vi "17.3 OCR Training.vi"() -> ()   [LabVIEW 2017]
uses:
  <vilib>/vision/OCR.llb/IMAQ OCR Threshold Mode.ctl
  <vilib>/vision/OCR.llb/IMAQ OCR Property.ctl
  <vilib>/vision/NI_Vision_Development_Module.lvlib
panel:
  out "Image":T1(plugin-control)
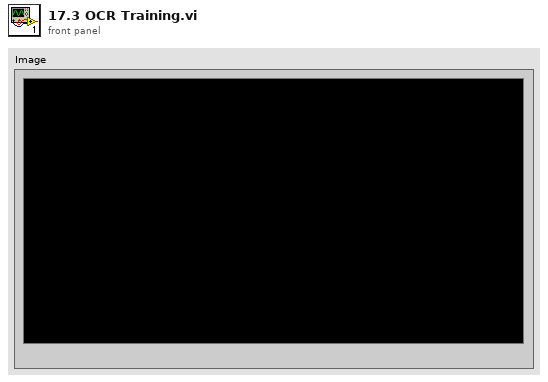
[diagram p1: front panel]
types:
  T1 = typedef "IMAQ Image.ctl" = refnum<image>
  T2 = typedef "IMAQ Rectangle" = cluster{"Left":i32, "Top":i32, "Right":i32, "Bottom":i32, "Rotation":dbl}
  T3 = typedef "IMAQ OCR Property.ctl" = i32
  T4 = cluster{"Dark Characters":bool, "Number of Blocks":i32, "Threshold Limits":cluster{"Lower Value":i32, "Upper Value":i32}, "Optimize For Speed":bool, "Perform Bi-modal Calculation":bool}
  T5 = typedef "IMAQ OCR Threshold Mode.ctl" = i32
  T6 = typedef "IMAQ OCR Session.ctl" = refnum<k1>
  T7 = typedef "ROI Descriptor" = cluster{"Global Rectangle":i32[], "Contours":cluster{"ID":enum32{"External", "Internal"}, "Type":u32, "Coordinates":i32[]}[]}
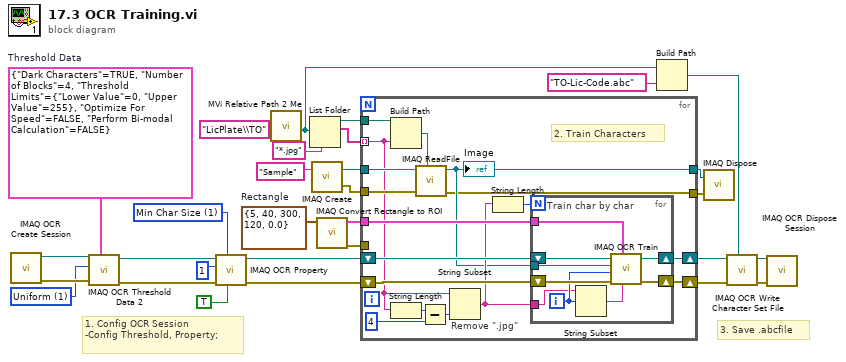
[diagram p0: block diagram]
diagram:
  w6 = T2 {"Left"=5, "Top"=40, "Right"=300, "Bottom"=120, "Rotation"=0.0}  # Rectangle
  w12 = T3 1 items=["Acceptance Level", "Min Char Size", "Max Char Size", "Min Char Spacing", "Max Horiz Element Spacing", "Max Vert Element Spacing", "Min Bounding Rect Width", "Max Bounding Rect Width", "Min Bounding Rect Height", "Max Bounding Rect Height", "Read Strategy", "Aspect Ratio", "Number Of Erosions", "Read Resolution", "Size of Char Set", "Substitution Character", "Remove Particles Touching ROI", "Auto Split", "Threshold Type", "Text Detection", "Line Separator", "Shortest Path Segment", "Min Pixels for Space"] ("Property")
  w16 = T4 {"Dark Characters"=TRUE, "Number of Blocks"=4, "Threshold Limits"={"Lower Value"=0, "Upper Value"=255}, "Optimize For Speed"=FALSE, "Perform Bi-modal Calculation"=FALSE}  # Threshold Data
  w19 = T5 1 items=["Fixed Range", "Uniform", "Linear", "Non-Linear"] ("Threshold Mode")
  # "3. Save .abcfile"
  # "1. Config OCR Session\n-Config Threshold, Property;"
  n1 = call "IMAQ OCR Create Session"() -> ("error out"=w20:errorcluster, "IMAQ OCR Session"=w21:T6)  [unwired: 10 in]
  n2 = call-poly "IMAQ OCR Threshold Data 2"("Threshold Data"=w16, "error in (no error)"=w20, "Threshold Mode"=w19, "IMAQ OCR Session"=w21) -> ("error out"=w17:errorcluster, "IMAQ OCR Session (dup)"=w18:T6)  [unwired: 3 in, 3 out]
  n3 = call-poly "IMAQ OCR Property"("Get/Set (True: Set)"=TRUE, "Property"=w12, "error in (no error)"=w17, "Property Value"=1, "IMAQ OCR Session"=w18) -> ("error out"=w15:errorcluster, "IMAQ OCR Session (dup)"=w14:T6)  [unwired: 4 in, 1 out]
  n4 = call "MVi Relative Path 2 Me.vi"("Relative Path"="LicPlate\\TO") -> ("Appended Dir"=w23:path)  [unwired: 5 in, 1 out]
  n5 = List Folder(path=w23, pattern="*.jpg") -> (path out=w25:path, filenames=w28:string[])  [unwired: 2 in, 2 out]
  n6 = call "IMAQ Create"("Image Name"="Sample") -> ("New Image"=w26:T1, "error out"=w24:errorcluster)  [unwired: 4 in]
  n7 = call "IMAQ Convert Rectangle to ROI"("Rectangle"=w6) -> ("error out"=w4:errorcluster, "ROI Descriptor"=w5:T7)  [unwired: 8 in]
  n8 = for {
    tunnel: w28 -> [w35] mode=indexing
    tunnel: w26 -> [w43]
    tunnel: w25 -> [w44]
    shift-right: [w38] -> w11
    shift-left: w15 -> [w40]
    tunnel: w24 -> [w42]
    shift-right: [w37] -> w10
    shift-left: w14 -> [w39]
    tunnel: w5 -> [w36]
    tunnel: w4 -> [_]
    tunnel: [w32] -> w2
    tunnel: [w31] -> w1
    # "2. Train Characters"
    # "Remove \".jpg\""
    n9 = Build Path(base path=w44, name or relative path=w35) -> (appended path=w41:path)
    n10 = String Length(string=w35) -> (length=w47:i32)
    n11 = call "IMAQ ReadFile"("File Path"=w41, "error in (no error)"=w42, "Image"=w43) -> ("error out"=w31:errorcluster, "Image Out"=w32:T1)  [unwired: 4 in, 3 out]
    "Image" <- w32
    n12 = Subtract(x=w47, y=4) -> (x-y=w45:i32)
    n13 = String Subset(string=w35, length (rest)=w45) -> (substring=w34:string)  [unwired: 1 in]
    n14 = String Length(string=w34) -> (length=w33:i32)
    n15 = for {
      N: w33 -> [_]
      tunnel: w36 -> [w52]
      shift-right: [w54] -> w38
      shift-left: w40 -> [w56]
      shift-right: [w53] -> w37
      shift-left: w39 -> [w55]
      tunnel: w34 -> [w50]
      tunnel: w32 -> [w48]
      i -> [w51]
      # "Train char by char"
      n16 = String Subset(string=w50, offset (0)=w51) -> (substring=w49:string)  [unwired: 1 in]
      n17 = call "IMAQ OCR Train"("Character Value"=w49, "ROI Descriptor"=w52, "error in (no error)"=w56, "Object Index"=w51, "Image"=w48, "IMAQ OCR Session"=w55) -> ("error out"=w54:errorcluster, "IMAQ OCR Session (dup)"=w53:T6)  [unwired: 3 in, 1 out]
    }
  }
  n18 = Build Path(base path=w23, name or relative path="TO-Lic-Code.abc" ("pattern")) -> (appended path=w9:path)
  n19 = call "IMAQ Dispose"("Image"=w2, "error in (no error)"=w1) -> ()  [unwired: 4 in, 1 out]
  n20 = call "IMAQ OCR Write Character Set File"("File Path"=w9, "error in (no error)"=w11, "IMAQ OCR Session"=w10) -> ("error out"=w8:errorcluster, "IMAQ OCR Session (dup)"=w7:T6)  [unwired: 7 in]
  n21 = call "IMAQ OCR Dispose Session"("error in (no error)"=w8, "IMAQ OCR Session"=w7) -> ()  [unwired: 9 in, 1 out]
